vi "Channel Power Enable.vi"(7 "All Channels (F)":bool, 8 "error in (no error)":errorcluster, 9 "Enable (OFF)":bool, 10 "Channel (0)":u8, 11 "BoardHandle":T1) -> (0 "error out":errorcluster, 3 "BoardHandle out":T1)   [LabVIEW 2020, in "CAEN PSM.lvlib"]
doc: "Enables or disables the output of the power supply."
uses:
  CAEN PSM.lvlib
  BoardHandle.ctl
  DeviceFamily.ctl
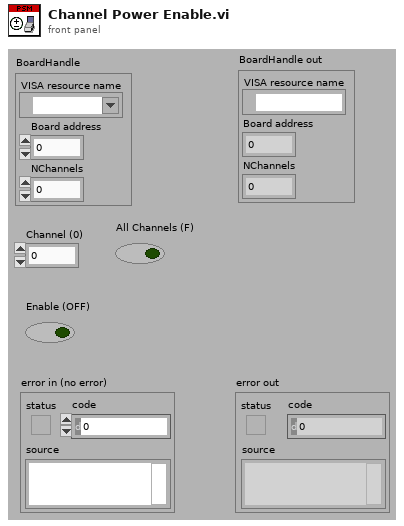
[diagram p1: front panel]
types:
  T1 = typedef "CAEN PSM.lvlib/BoardHandle.ctl" = cluster{"VISA resource name":refnum<visa-resource-name>, "Board address":i8, "NChannels":u8}
  T2 = typedef "CAEN PSM.lvlib/DeviceFamily.ctl" = enum8{"NIM / DESKTOP HV", "DT55XXE HV", "SMART HV"}
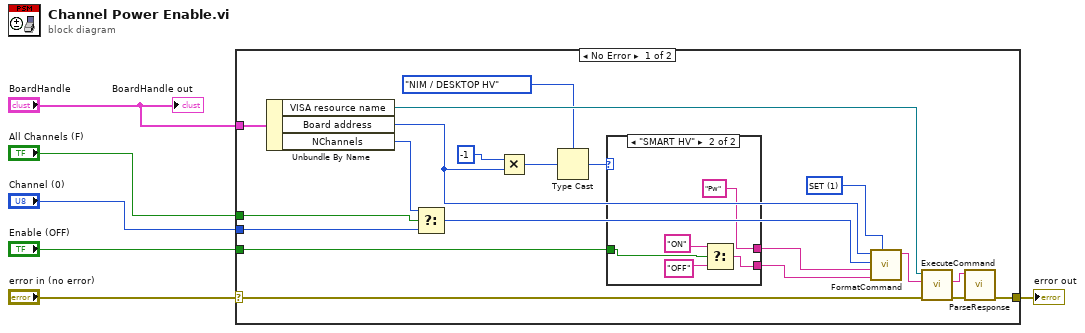
[diagram p0: block diagram]
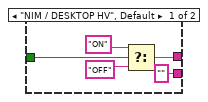
[diagram p2: hidden frame]
diagram:
  n1 = case shown="No Error" "error in (no error)" {
    selector: "error in (no error)" -> [w13 w37]
    tunnel: "Enable (OFF)" -> [w26 _]
    tunnel: "All Channels (F)" -> [w23 _]
    tunnel: "Channel (0)" -> [w21 _]
    tunnel: [w16 w37] -> w3
    tunnel: "BoardHandle" -> [w14 _]
    frame No Error {
      w24 = u8 1 items=["MON", "SET"] ("CMD")
      n2 = Unbundle By Name(w14) -> ("VISA resource name"=w19:refnum<visa-resource-name>, "Board address"=w9:i8, "NChannels"=w22:u8)
      n3 = Select(t=w22, s=w23, f=w21) -> (s? t:f=w20:u8)
      n4 = Multiply(x=i8 -1, y=w9) -> (x*y=w12:i8)
      n5 = Type Cast(type=DeviceFamily."NIM / DESKTOP HV" ("Device Family"), x=w12) -> (*(type *) &x=w8:T2)
      n6 = case shown="\"SMART HV\"" w8 {
        tunnel: w26 -> [w31 w32]
        tunnel: [w28 "Pw"] -> w25
        tunnel: ["" w33] -> w7
        frame "NIM / DESKTOP HV", Default {
          n7 = Select(t="ON", s=w31, f="OFF") -> (s? t:f=w28:string)
        }
        frame "SMART HV" {
          n8 = Select(t="ON", s=w32, f="OFF") -> (s? t:f=w33:string)
        }
      }
      n9 = call "FormatCommand.vi"("CMD (MON)"=w24, "VAL"=w7, "PAR"=w25, "CH"=w20, "BD (0)"=w9) -> ("cmd"=w18:string)  [unwired: 6 in]
      n10 = call "ExecuteCommand.vi"("error in (no error)"=w13, "Command"=w18, "VISA resource name"=w19) -> ("error out"=w17:errorcluster, "Response"=w15:string)  [unwired: 6 in, 1 out]
      n11 = call "ParseResponse.vi"("error in (no error)"=w17, "Response"=w15) -> ("error out"=w16:errorcluster)  [unwired: 6 in, 3 out]
    }
    frame Error {
    }
  }
  "error out" <- w3
  "BoardHandle out" <- "BoardHandle"
